vi "serialization test.vi"() -> ()   [LabVIEW 2013, in "NISE_CEF_Tests.lvlib"]
uses:
  NISE_CEF_Tests.lvlib
  Trunk/CEF_TreeControl/serializable configuration/NISE_CEF_serializable configuration.lvclass
  Trunk/CEF_TreeControl/serializable configuration/NISE_CEF_serializable configuration.lvclass/NISE_CEF_serializable configuration.ctl
panel:
  out "serOK":bool
  out "keys ok":bool
  out "class identical":bool
  out "name ok":bool
  out "no error":errorcluster
  out "version ok":bool
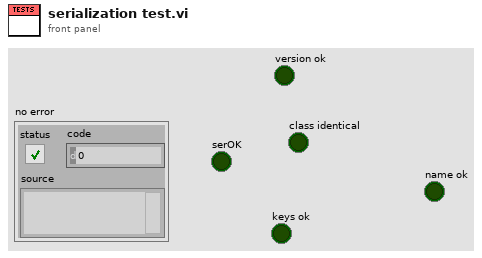
[diagram p1: front panel]
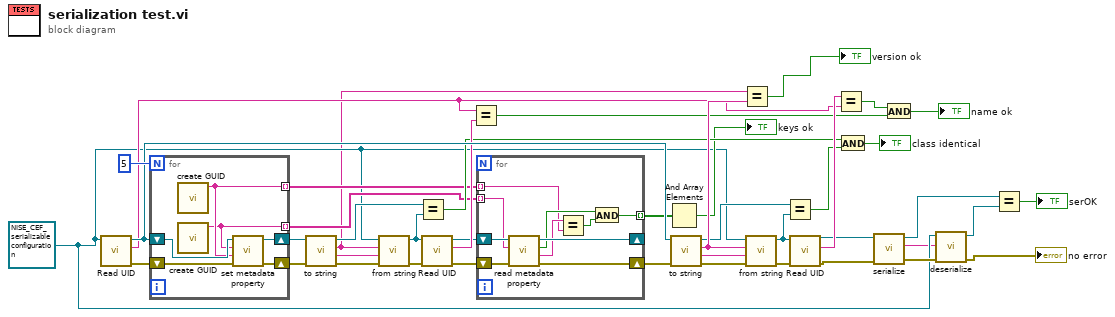
[diagram p0: block diagram]
diagram:
  w8 = refnum<class "NISE_CEF_serializable configuration.lvclass"> refnum ("configuration")
  n1 = call "Read UID.vi"("configuration in"=w8) -> ("error out"=w36:errorcluster, "instance id"=w28:string, "configuration out"=w37:refnum<class "NISE_CEF_serializable configuration.lvclass">)  [unwired: 8 in]
  n2 = for {
    N: 5 -> [_]
    shift-right: [w48] -> w27
    shift-left: w37 -> [w49]
    shift-right: [w47] -> w33
    shift-left: w36 -> [w46]
    tunnel: [w45] -> w17 mode=indexing
    tunnel: [w44] -> w18 mode=indexing
    n3 = call "create GUID.vi"() -> ("uuid"=w45:string)  [unwired: 11 in]
    n4 = call "create GUID.vi"() -> ("uuid"=w44:string)  [unwired: 11 in]
    n5 = call "set metadata property.vi"("error in"=w46, "value"=w45, "key"=w44, "configuration in"=w49) -> ("error out"=w47:errorcluster, "configuration out"=w48:refnum<class "NISE_CEF_serializable configuration.lvclass">)  [unwired: 6 in]
  }
  n6 = call-dynamic "to string.vi"("error in"=w33, "configuration in"=w27) -> ("error out"=w34:errorcluster, "data"=w35:string, "version"=w1:string, "configuration out"=w24:refnum<class "NISE_CEF_serializable configuration.lvclass">)  [unwired: 6 in]
  n7 = call-dynamic "from string.vi"("error in"=w34, "data"=w35, "version"=w1, "configuration in"=w8) -> ("error out"=w30:errorcluster, "configuration out"=w26:refnum<class "NISE_CEF_serializable configuration.lvclass">)  [unwired: 6 in]
  n8 = Equal?(x=w24, y=w26) -> (x = y?=w19:bool)
  n9 = call "Read UID.vi"("error in"=w30, "configuration in"=w26) -> ("error out"=w15:errorcluster, "instance id"=w29:string, "configuration out"=w16:refnum<class "NISE_CEF_serializable configuration.lvclass">)  [unwired: 7 in]
  n10 = Equal?(x=w28, y=w29) -> (x = y?=w22:bool)
  n11 = for {
    tunnel: w18 -> [w55] mode=indexing
    tunnel: w17 -> [w52] mode=indexing
    shift-right: [w57] -> _
    shift-left: w16 -> [w58]
    shift-right: [w56] -> w14
    shift-left: w15 -> [w59]
    tunnel: [w50] -> w13 mode=indexing
    n12 = call "read metadata property.vi"("error in"=w59, "key"=w55, "configuration in"=w58) -> ("error out"=w56:errorcluster, "value"=w53:string, "found"=w54:bool, "configuration out"=w57:refnum<class "NISE_CEF_serializable configuration.lvclass">)  [unwired: 5 in]
    n13 = Equal?(x=w53, y=w52) -> (x = y?=w51:bool)
    n14 = And(x=w54, y=w51) -> (x .and. y?=w50:bool)
  }
  n15 = And Array Elements(Boolean array=w13) -> (logical AND=→"keys ok":bool)
  n16 = call-dynamic "to string.vi"("error in"=w14, "configuration in"=w37) -> ("error out"=w43:errorcluster, "data"=w39:string, "version"=w42:string, "configuration out"=w25:refnum<class "NISE_CEF_serializable configuration.lvclass">)  [unwired: 6 in]
  n17 = Equal?(x=w1, y=w42) -> (x = y?=→"version ok":bool)
  n18 = call-dynamic "from string.vi"("error in"=w43, "data"=w39, "version"=w42, "configuration in"=w8) -> ("error out"=w41:errorcluster, "configuration out"=w23:refnum<class "NISE_CEF_serializable configuration.lvclass">)  [unwired: 6 in]
  n19 = Equal?(x=w25, y=w23) -> (x = y?=w20:bool)
  n20 = call "Read UID.vi"("error in"=w41, "configuration in"=w23) -> ("error out"=w7:errorcluster, "instance id"=w40:string, "configuration out"=w9:refnum<class "NISE_CEF_serializable configuration.lvclass">)  [unwired: 7 in]
  n21 = Equal?(x=w40, y=w28) -> (x = y?=w31:bool)
  n22 = And(x=w19, y=w20) -> (x .and. y?=→"class identical":bool)
  n23 = call "serialize.vi"("error in"=w7, "configuration in"=w9) -> ("error out"=w10:errorcluster, "serialized form"=w5:string, "configuration out"=w3:refnum<class "NISE_CEF_serializable configuration.lvclass">)  [unwired: 7 in]
  n24 = And(x=w31, y=w22) -> (x .and. y?=→"name ok":bool)
  n25 = call "deserialize.vi"("error in"=w10, "serialized form"=w5, "configuration in"=w8) -> ("error out"=→"no error":errorcluster, "configuration out"=w4:refnum<class "NISE_CEF_serializable configuration.lvclass">)  [unwired: 7 in]
  n26 = Equal?(x=w3, y=w4) -> (x = y?=→"serOK":bool)
